vi "move Y Relative.vi"(9 "Settings":T1, 10 "Y Speed":u32, 11 "y mm":dbl) -> ()   [LabVIEW 2017]
uses:
  Settings/Settings-Control.ctl
  ICNC/ICNC2.lvlib
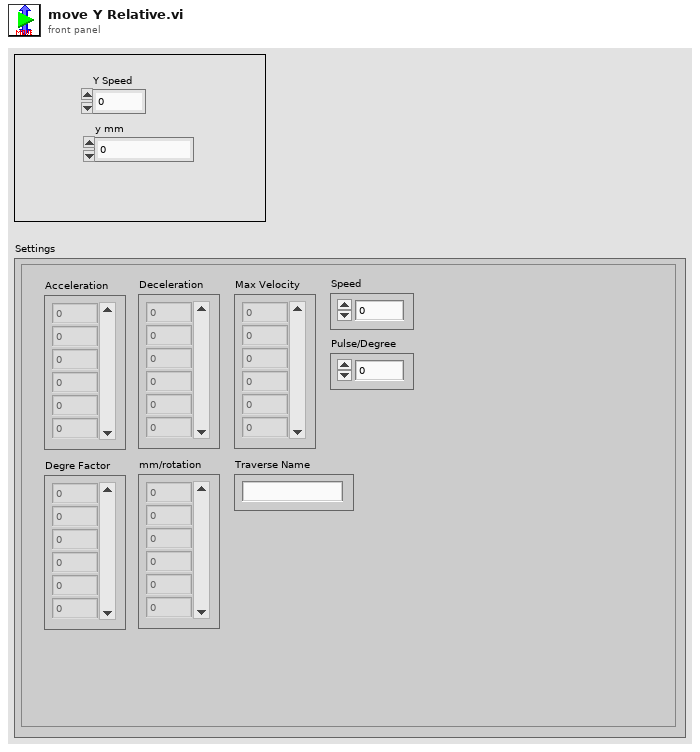
[diagram p1: front panel]
types:
  T1 = typedef "Settings-Control.ctl" = cluster{"Acceleration":dbl[], "Deceleration":dbl[], "Max Velocity":dbl[], "Speed":dbl, "Pulse/Degree":dbl, "Degre Factor":dbl[], "mm/rotation":dbl[], "Traverse Name":string}
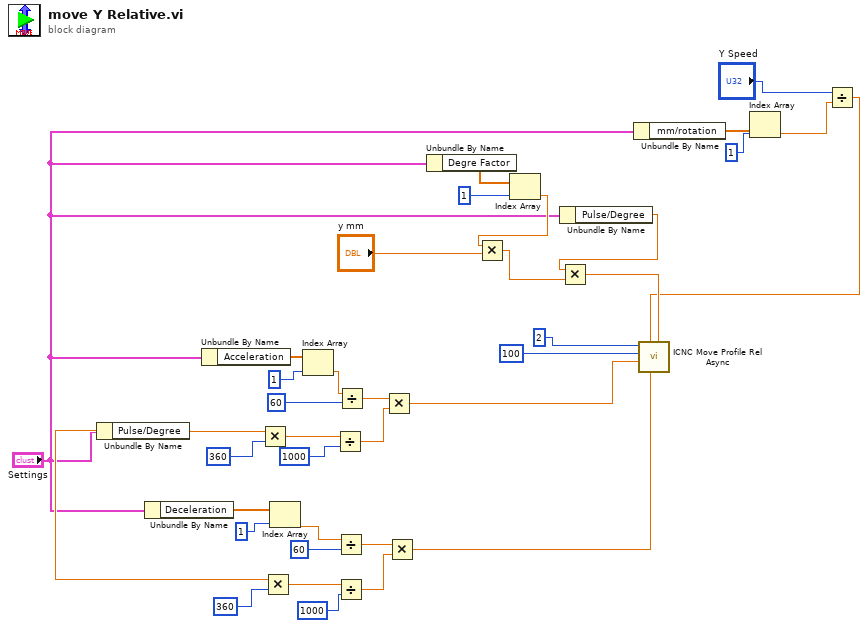
[diagram p0: block diagram]
diagram:
  n1 = Unbundle By Name("Settings") -> ("Pulse/Degree"=w18:dbl)
  n2 = Unbundle By Name("Settings") -> ("Deceleration"=w14:dbl[])
  n3 = Unbundle By Name("Settings") -> ("Acceleration"=w17:dbl[])
  n4 = Multiply(x=w18, y=360) -> (x*y=w26:dbl)
  n5 = Multiply(x=w18, y=360) -> (x*y=w25:dbl)
  n6 = Index Array(array=w14, index=1) -> (element=w13:dbl)
  n7 = Index Array(array=w17, index=1) -> (element=w15:dbl)
  n8 = Divide(x=w26, y=1000) -> (x/y=w36:dbl)
  n9 = Divide(x=w13, y=60) -> (x/y=w32:dbl)
  n10 = Divide(x=w25, y=1000) -> (x/y=w31:dbl)
  n11 = Divide(x=w15, y=60) -> (x/y=w27:dbl)
  n12 = Multiply(x=w27, y=w36) -> (x*y=w22:dbl)
  n13 = Multiply(x=w32, y=w31) -> (x*y=w21:dbl)
  n14 = Unbundle By Name("Settings") -> ("Degre Factor"=w10:dbl[])
  n15 = Index Array(array=w10, index=1) -> (element=w8:dbl)
  n16 = Multiply(x=w8, y="y mm") -> (x*y=w20:dbl)
  n17 = Unbundle By Name("Settings") -> ("Pulse/Degree"=w9:dbl)
  n18 = Multiply(x=w9, y=w20) -> (x*y=w19:dbl)
  n19 = Unbundle By Name("Settings") -> ("mm/rotation"=w6:dbl[])
  n20 = Index Array(array=w6, index=1) -> (element=w4:dbl)
  n21 = Divide(x="Y Speed", y=w4) -> (x/y=w2:dbl)
  n22 = call <userlib>:"ICNC Move Profile Rel Async.vi"("Distance"=w19, "Decel"=w21, "Speed"=w2, "Accel"=w22, "FStartStop"=100, "Axe"=2) -> ()  [unwired: 4 in, 2 out]
